vi "小时数据主动发送(子VI).vi"   [LabVIEW 2016]
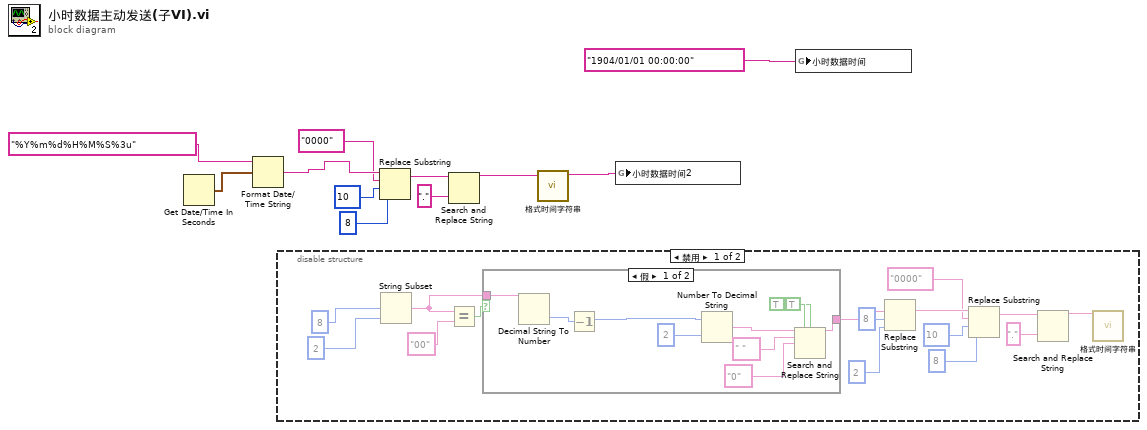
[diagram p0: block diagram]
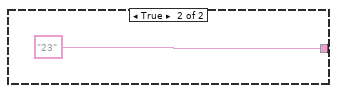
[diagram p2: hidden frame]
diagram:
  n1 = Get Date/Time In Seconds() -> (seconds since 1Jan1904=w8:timestamp)
  n2 = Format Date/Time String(time format string (%c)="%Y%m%d%H%M%S%3u" ("时间格式字符串(%c)"), seconds (now)=w8) -> (date/time string=w11:string)  [unwired: 1 in]
  n3 = disable-structure shown="禁用" {
    frame Disabled {
      n4 = String Subset(offset (0)=8 ("偏移量(0)"), length (rest)=2 ("长度（子字符串长度）")) -> (string=w12:string, substring=w18:string)
      n5 = Equal?(x=w18, y="00") -> (x = y?=w17:bool)
      n6 = case shown="假" w17 {
        tunnel: w18 -> [w38 _]
        tunnel: [w30 "23" ("y")] -> w19
        frame False {
          n7 = Decimal String To Number(string=w38) -> (number=w37:i32)  [unwired: 2 in, 1 out]
          n8 = Decrement(x=w37) -> (x-1=w31:i32)
          n9 = Number To Decimal String(number=w31, width (-)=i16 2 ("宽度(-)")) -> (decimal integer string=w33:string)
          n10 = Search and Replace String(replace all?=TRUE ("替换全部？(F)"), case sensitive?=TRUE ("忽略大小写？(F)"), input string=w33, search string=" " ("搜索字符串"), replace string="0" ("替换字符串(\"\")")) -> (result string=w30:string)  [unwired: 3 in, 3 out]
        }
        frame True {
        }
      }
      n11 = Replace Substring(2:2 ("长度（子字符串长度）"), 3:8 ("偏移量(0)"), 4:w19) -> (1:w28:string, 5:w13:string)  [unwired: 1 out]
      n12 = Replace Substring(2:8 ("长度（子字符串长度）"), 3:10 ("偏移量(0)"), 4:"0000" ("子字符串(\"\")"), 5:w28) -> (1:w24:string)  [unwired: 1 out]
      n13 = Search and Replace String(input string=w24, search string="." ("搜索字符串")) -> (result string=w22:string)  [unwired: 6 in, 3 out]
      n14 = call "格式时间字符串.vi"("字符串"=w22) -> ()  [unwired: 10 in, 1 out]
    }
    frame Enabled {
    }
  }
  n15 = Replace Substring(2:8 ("长度（子字符串长度）"), 3:10 ("偏移量(0)"), 4:"0000" ("子字符串(\"\")"), 5:w11) -> (1:w6:string)  [unwired: 1 out]
  n16 = Search and Replace String(input string=w6, search string="." ("搜索字符串")) -> (result string=w10:string)  [unwired: 6 in, 3 out]
  n17 = call "格式时间字符串.vi"("字符串"=w10) -> ("连接的字符串"=w2:string)  [unwired: 10 in]
  n18 = global write "全局 时间2.vi" "小时数据时间2"(w2) -> ()
  n19 = global write "全局 时间.vi" "小时数据时间"("1904/01/01 00:00:00") -> ()
